vi "fyp (2) (1).vi"() -> ()   [LabVIEW 2021]
uses:
  <vilib>/userDefined/High Color/IMAQdx.ctl
  <vilib>/vision/driver/IMAQdx.llb/IMAQdx Camera Control Mode.ctl
  <vilib>/vision/driver/IMAQdx.llb/IMAQdx Acquisition Mode.ctl
  <vilib>/vision/driver/IMAQdx.llb/IMAQdx Buffer Number Mode.ctl
  <vilib>/vision/Management.llb/Cast Image 2 Method.ctl
  <vilib>/myRIO/Instrument Drivers/Onboard IO/PWM/typedefs/PWM Reference.ctl
  <vilib>/myRIO/Common/Instrument Driver Framework/Utilities/typedefs/myRIO Generic Hardware Reference.ctl
  <vilib>/myRIO/Common/Instrument Driver Framework/Utilities/typedefs/Hardware Version Enum.ctl
  <vilib>/myRIO/Common/Instrument Driver Framework/Utilities/typedefs/myRIO v1.0 Reference.ctl
  <vilib>/myRIO/Common/Instrument Driver Framework/Utilities/typedefs/Generic FPGA Reference.ctl
  <vilib>/myRIO/Common/Instrument Driver Framework/myRIO v1.0/PWM/typedefs/PWM Channels Enum.ctl
  <vilib>/myRIO/Instrument Drivers/Onboard IO/PWM/typedefs/PWM Configuration.ctl
  <vilib>/userDefined/High Color/nirio_resource_hc.ctl
  <vilib>/myRIO/Instrument Drivers/Onboard IO/DIO/typedefs/DIO Reference.ctl
  <vilib>/myRIO/Common/Instrument Driver Framework/myRIO v1.0/DIO/typedefs/DIO Channels List.ctl
  <vilib>/myRIO/Common/Instrument Driver Framework/myRIO v1.0/DIO/typedefs/DIO Channels Enum.ctl
  <vilib>/myRIO/Instrument Drivers/Onboard IO/AI/typedefs/AI Reference.ctl
  <vilib>/myRIO/Common/Instrument Driver Framework/myRIO v1.0/AI/typedefs/AI Channels List.ctl
  <vilib>/myRIO/Common/Instrument Driver Framework/myRIO v1.0/AI/typedefs/AI Channels Enum.ctl
  <vilib>/myRIO/Common/Instrument Driver Framework/Utilities/typedefs/Analog Scaling Constants List.ctl
  <vilib>/myRIO/Common/Instrument Driver Framework/Utilities/typedefs/Analog Scaling Constants.ctl
  <vilib>/myRIO/Common/Instrument Driver Framework/myRIO v1.0/DIO/vis/myRIO v1.1 Open DIO.vi
  <vilib>/myRIO/Common/Instrument Driver Framework/myRIO v1.0/PWM/vis/myRIO v1.1 Open PWM.vi
  <vilib>/myRIO/Common/Instrument Driver Framework/myRIO v1.0/AI/vis/myRIO v1.1 Open AI.vi
  <vilib>/myRIO/Common/Instrument Driver Framework/Utilities/vis/Validate Channels.vi
  <vilib>/myRIO/Common/Instrument Driver Framework/myRIO v1.0/DIO/vis/myRIO v1.0 Reserve DIO.vi
  <vilib>/myRIO/Common/Instrument Driver Framework/myRIO v1.0/PWM/vis/myRIO v1.0 Reserve PWM.vi
  <vilib>/myRIO/Instrument Drivers/Onboard IO/PWM/vis/Set Duty Cycle and Frequency.vi
  <vilib>/myRIO/Common/Instrument Driver Framework/myRIO v1.0/PWM/vis/myRIO v1.0 Close PWM.vi
  <vilib>/myRIO/Common/Instrument Driver Framework/myRIO v1.0/DIO/vis/myRIO v1.0 Close DIO.vi
  <vilib>/myRIO/Common/Instrument Driver Framework/myRIO v1.0/AI/vis/myRIO v1.0 Reserve AI.vi
  <vilib>/myRIO/Common/Instrument Driver Framework/myRIO v1.0/AI/vis/myRIO v1.0 Close AI.vi
  <vilib>/myRIO/Common/Instrument Driver Framework/myRIO v1.0/Resource Manager/vis/myRIO v1.0 Reserve Channel List.vi
  <vilib>/myRIO/Common/Instrument Driver Framework/myRIO v1.0/DIO/vis/myRIO v1.0 Build MUX Configuration DIO.vi
  <vilib>/myRIO/Common/Instrument Driver Framework/myRIO v1.0/PWM/vis/myRIO v1.0 Build MUX Configuration PWM.vi
  <vilib>/myRIO/Common/Instrument Driver Framework/myRIO v1.0/PWM/vis/myRIO v1.0 Unreserve PWM.vi
  <vilib>/myRIO/Common/Instrument Driver Framework/myRIO v1.0/DIO/vis/myRIO v1.0 Unreserve DIO.vi
  <vilib>/myRIO/Common/Instrument Driver Framework/myRIO v1.0/AI/vis/myRIO v1.0 Build MUX Configuration AI.vi
  <vilib>/myRIO/Common/Instrument Driver Framework/myRIO v1.0/AI/vis/myRIO v1.0 Unreserve AI.vi
  <vilib>/myRIO/Common/Instrument Driver Framework/myRIO v1.0/Resource Manager/vis/myRIO v1.0 Reserve Channel.vi
  <vilib>/myRIO/Common/Instrument Driver Framework/myRIO v1.0/Resource Manager/vis/myRIO v1.0 Unreserve Channel.vi
  <vilib>/myRIO/Common/Instrument Driver Framework/myRIO v1.0/Resource Manager/vis/myRIO v1.0 Create Configuration List.vi
  <vilib>/myRIO/Common/Instrument Driver Framework/myRIO v1.0/Resource Manager/vis/myRIO v1.0 Unreserve Channel List.vi
  <vilib>/myRIO/Common/Instrument Driver Framework/myRIO v1.0/Resource Manager/vis/myRIO v1.0 Build Mutex Name.vi
  <vilib>/Utility/VariantDataType/GetNumericInfo.vi
  <vilib>/Utility/error.llb/Error Cluster From Error Code.vi
  <vilib>/myRIO/Common/Instrument Driver Framework/myRIO v1.0/myRIO v1.1 Open.vi
  <vilib>/myRIO/Common/Instrument Driver Framework/myRIO v1.0/AI/vis/myRIO v1.0 Get Scaling Constants AI.vi
  <vilib>/myRIO/Common/Instrument Driver Framework/Utilities/vis/IO Manager.vi
  <vilib>/myRIO/Common/Instrument Driver Framework/Utilities/vis/Configuration Manager.vi
  <vilib>/myRIO/Common/Instrument Driver Framework/myRIO v1.0/myRIO v1.0 Close.vi
  <vilib>/myRIO/Common/Instrument Driver Framework/myRIO v1.0/Resource Manager/vis/myRIO v1.0 Configure IO.vi
  <vilib>/myRIO/Common/Instrument Driver Framework/myRIO v1.0/PWM/vis/myRIO v1.0 Write PWM.vi
  <vilib>/myRIO/Common/Instrument Driver Framework/myRIO v1.0/DIO/vis/myRIO v1.0 Read DIO.vi
  <vilib>/myRIO/Common/Instrument Driver Framework/myRIO v1.0/PWM/vis/myRIO v1.0 Shutdown PWM.vi
  <vilib>/myRIO/Common/Instrument Driver Framework/myRIO v1.0/DIO/vis/myRIO v1.0 Shutdown DIO.vi
  <vilib>/myRIO/Common/Instrument Driver Framework/myRIO v1.0/DIO/vis/myRIO v1.0 Write DIO.vi
  <vilib>/myRIO/Common/Instrument Driver Framework/myRIO v1.0/AI/vis/myRIO v1.0 Read AI.vi
  <vilib>/myRIO/Instrument Drivers/Onboard IO/AI/vis/myRIO AI Open.xnode
  <vilib>/myRIO/Instrument Drivers/Onboard IO/DIO/vis/myRIO DIO Open.xnode
  <vilib>/myRIO/Instrument Drivers/Onboard IO/PWM/vis/myRIO PWM Open.xnode
  <vilib>/vision/driver/NI_Vision_Acquisition_Software.lvlib
  <vilib>/myRIO/Instrument Drivers/Onboard IO/DIO/DIO.lvlib
  <vilib>/myRIO/Instrument Drivers/Onboard IO/AI/AI.lvlib
  <vilib>/myRIO/Instrument Drivers/Onboard IO/PWM/PWM.lvlib
  <vilib>/vision/NI_Vision_Development_Module.lvlib
panel:
  out "error out 2":errorcluster
  in  "LED0":bool
  out "Image 2":T1(plugin-control)
  in  "Session In 2":T2
  out "Colour Match Score 2":i32[](array[numeric])
  out "Is Colour from Sample Detected 2":bool
  out "Number of Circles Returned 2":i32
  out "Boolean 4":bool
  in  "error in (no error)":errorcluster
  out "Boolean 2":bool
  in  "error in (no error) 3":errorcluster
  in  "error in (no error) 2":errorcluster
  out "error out":errorcluster
  out "Darkness level":dbl(slide) scale=0.0..1.0
  out "Numeric":dbl format="%.2f"
  out "Image":T1(plugin-control)
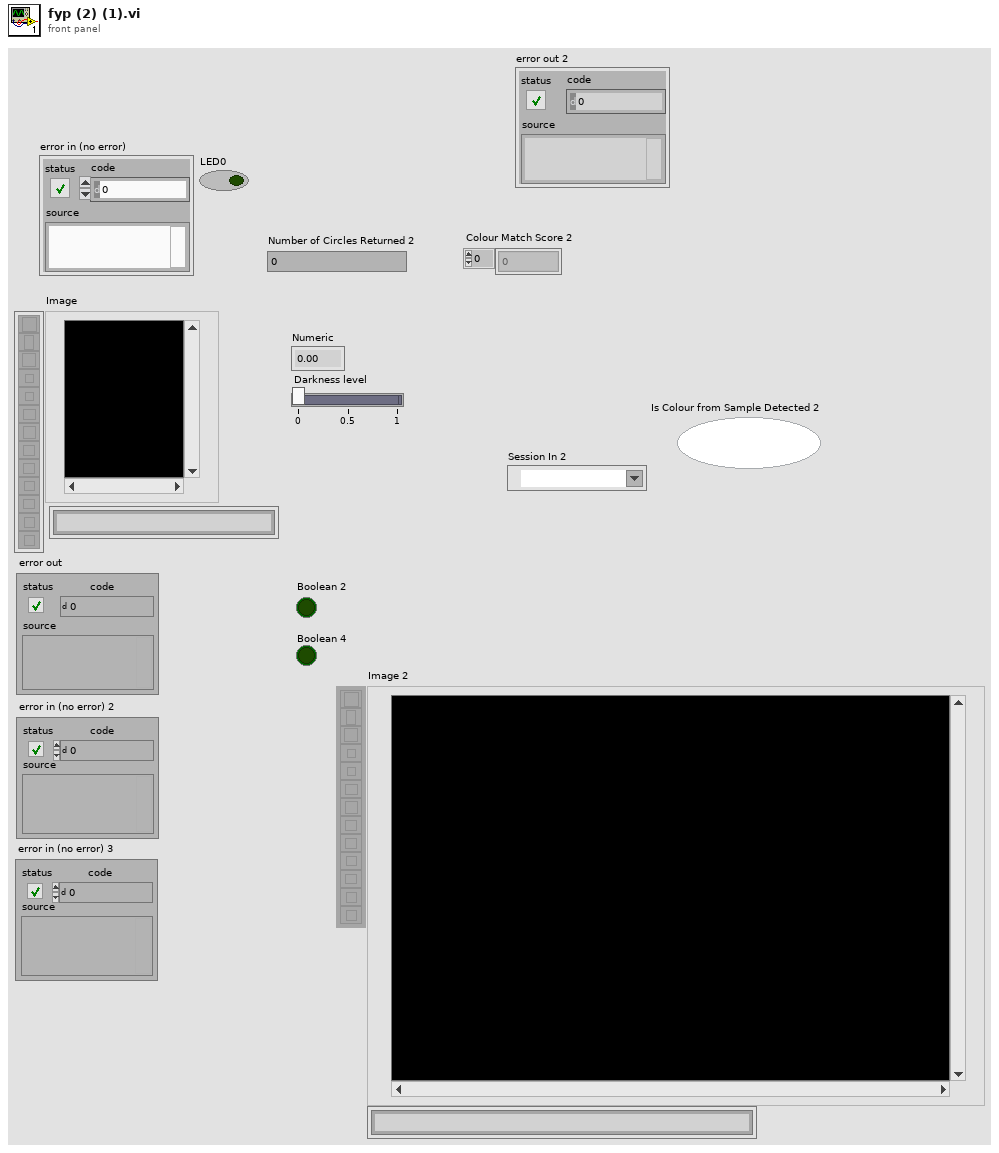
[diagram p1: front panel]
types:
  T1 = typedef "IMAQ Image.ctl" = refnum<image>
  T2 = typedef "IMAQdx.ctl" = refnum<k21>
  T3 = typedef "Cast Image 2 Method.ctl" = u32
  T4 = typedef "Image Type" = u32
  T5 = typedef "IMAQ Rectangle" = cluster{"Left":i32, "Top":i32, "Right":i32, "Bottom":i32, "Rotation":dbl}
  T6 = typedef "NI_Vision_Acquisition_Software.lvlib/IMAQdx Buffer Number Mode.ctl" = enum32{"Next", "Last", "Buffer Number", "Every", "Last New"}
  T7 = typedef "NI_Vision_Acquisition_Software.lvlib/IMAQdx Acquisition Mode.ctl" = enum32{"One Shot", "Continuous"}
  T8 = typedef "NI_Vision_Acquisition_Software.lvlib/IMAQdx Camera Control Mode.ctl" = enum32{"Controller", "Listener"}
  T9 = typedef "DIO.lvlib/DIO Reference.ctl" = cluster{"myRIO Reference":T10, "DIO Channels List":T14}
  T10 = typedef "myRIO Generic Hardware Reference.ctl" = cluster{"myRIO Model":T11, "myRIO Hardware Reference":T12}
  T11 = typedef "Hardware Version Enum.ctl" = enum16{"Unknown", "myRIO-1900", "myRIO-1950", "roboRIO", "NI ELVIS RIO CM", "ELVIS III"}
  T12 = typedef "myRIO v1.0 Reference.ctl" = cluster{"Generic FPGA Reference":T13, "Allow multiple opens":bool}
  T13 = typedef "Generic FPGA Reference.ctl" = refnum<k20>
  T14 = typedef "DIO Channels List.ctl" = T15[]
  T15 = typedef "DIO Channels Enum.ctl" = enum16{"Not Connected", "C/DIO0", "C/DIO1", "C/DIO2", "C/DIO3", "C/DIO4", "C/DIO5", "C/DIO6", "C/DIO7", "A/DIO0", "A/DIO1", "A/DIO2", "A/DIO3", "A/DIO4", "A/DIO5", "A/DIO6", "A/DIO7", "A/DIO8", "A/DIO9", "A/DIO10", "A/DIO11", "A/DIO12", "A/DIO13", "A/DIO14", "A/DIO15", "A/DIO16", "A/DIO17", "A/DIO18", "A/DIO19", "B/DIO0", "B/DIO1", "B/DIO2", "B/DIO3", "B/DIO4", "B/DIO5", "B/DIO6", "B/DIO7", "B/DIO8", "B/DIO9", "B/DIO10", "B/DIO11", "B/DIO12", "B/DIO13", "B/DIO14", "B/DIO15", "B/DIO16", "B/DIO17", "B/DIO18", "B/DIO19", "LED0", "LED1", "LED2", "LED3", "Button0", "DIO/DIO0", "DIO/DIO1", "DIO/DIO2", "DIO/DIO3", "DIO/DIO4", "DIO/DIO5", "DIO/DIO6", "DIO/DIO7", "DIO/DIO8", "DIO/DIO9", "SPI/CS0", "SPI/CS1", "SPI/CS2", "SPI/CS3", "LED RADIO (Green)", "LED RADIO (Red)", "LED COMM (Green)", "LED COMM (Red)", "LED MODE (Green)", "LED MODE (Red)"}
  T16 = typedef "PWM.lvlib/PWM Reference.ctl" = cluster{"myRIO Reference":T10, "PWM Channels Enum":T17, "PWM Configuration":T18}
  T17 = typedef "PWM Channels Enum.ctl" = enum16{"Not Connected", "C/PWM0", "C/PWM1", "A/PWM0", "A/PWM1", "A/PWM2", "A/PWM3", "A/PWM4", "A/PWM5", "A/PWM6", "A/PWM7", "A/PWM8", "A/PWM9", "A/PWM10", "A/PWM11", "A/PWM12", "A/PWM13", "A/PWM14", "A/PWM15", "A/PWM16", "A/PWM17", "A/PWM18", "A/PWM19", "B/PWM0", "B/PWM1", "B/PWM2", "B/PWM3", "B/PWM4", "B/PWM5", "B/PWM6", "B/PWM7", "B/PWM8", "B/PWM9", "B/PWM10", "B/PWM11", "B/PWM12", "B/PWM13", "B/PWM14", "B/PWM15", "B/PWM16", "B/PWM17", "B/PWM18", "B/PWM19", "PWM/PWM0", "PWM/PWM1", "PWM/PWM2", "PWM/PWM3", "PWM/PWM4", "PWM/PWM5", "PWM/PWM6", "PWM/PWM7", "PWM/PWM8", "PWM/PWM9"}
  T18 = typedef "PWM.lvlib/PWM Configuration.ctl" = cluster{"Frequency":dbl, "Duty Cycle":dbl}
  T19 = typedef "AI.lvlib/AI Reference.ctl" = cluster{"myRIO Reference":T10, "AI Channels List":T20, "AI Scaling Constants List":T22}
  T20 = typedef "AI Channels List.ctl" = T21[]
  T21 = typedef "AI Channels Enum.ctl" = enum16{"Not Connected", "AudioIn/Left", "AudioIn/Right", "C/AI0", "C/AI1", "A/AI0", "A/AI1", "A/AI2", "A/AI3", "A/AI4", "A/AI5", "A/AI6", "A/AI7", "B/AI0", "B/AI1", "B/AI2", "B/AI3", "B/AI4", "B/AI5", "B/AI6", "B/AI7", "AI/AI0", "AI/AI1", "AI/AI2", "AI/AI3", "A/AI0 (DIFF)", "A/AI1 (DIFF)", "A/AI2 (DIFF)", "A/AI3 (DIFF)", "B/AI0 (DIFF)", "B/AI1 (DIFF)", "B/AI2 (DIFF)", "B/AI3 (DIFF)"}
  T22 = typedef "Analog Scaling Constants List.ctl" = T23[]
  T23 = typedef "Analog Scaling Constants.ctl" = cluster{"LSB Weight (Volts)":dbl, "Offset (Volts)":dbl, "Signed?":bool}
  T24 = typedef "ROI Descriptor" = cluster{"Global Rectangle":i32[], "Contours":cluster{"ID":enum32{"External", "Internal"}, "Type":u32, "Coordinates":i32[]}[]}
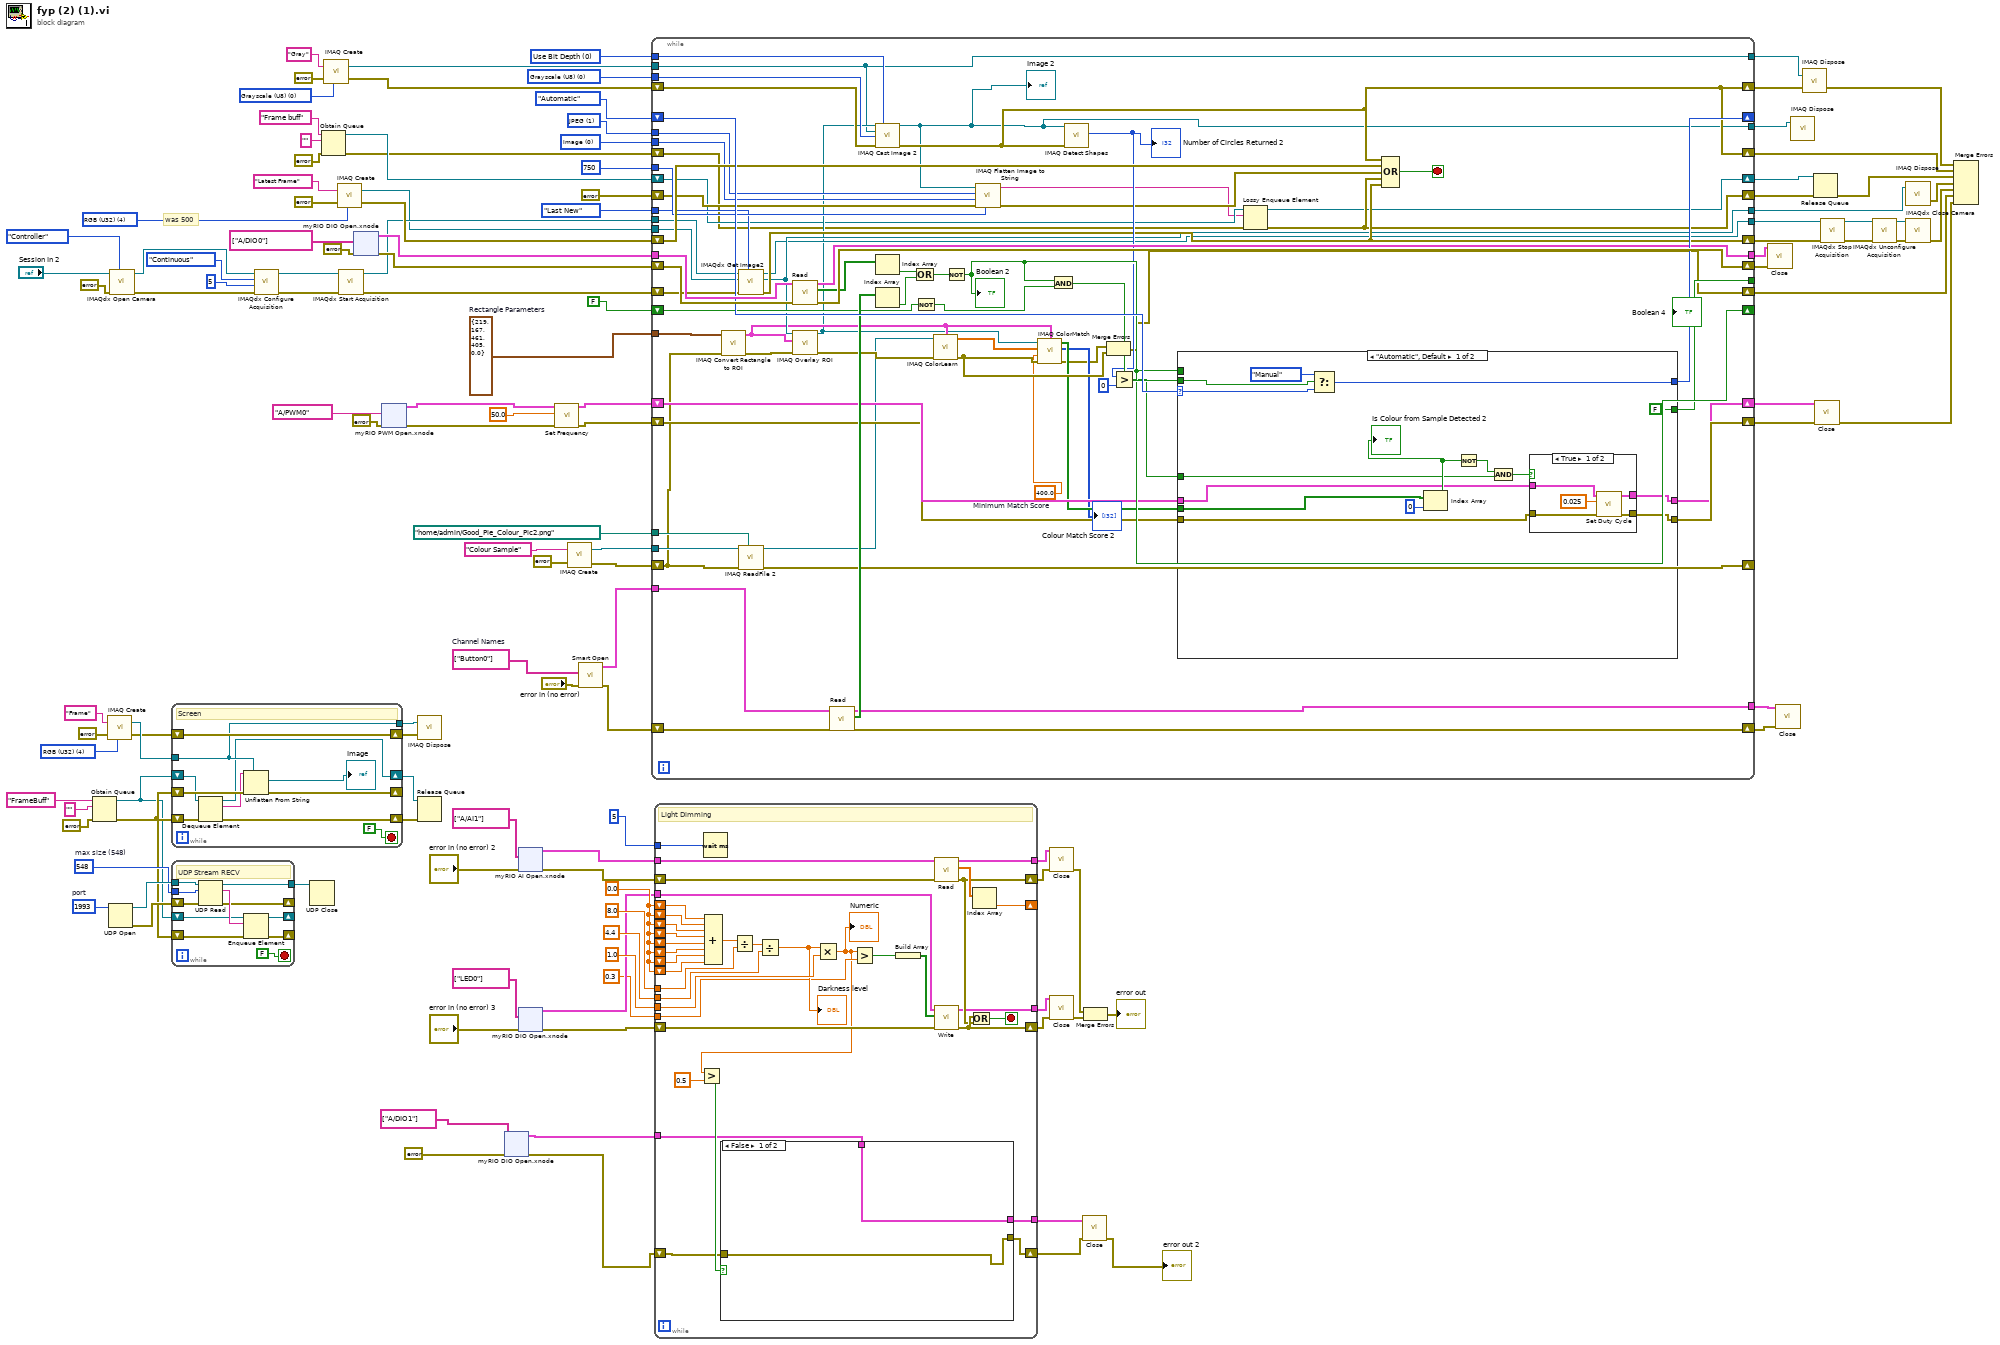
[diagram p0: block diagram]
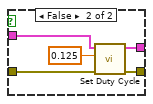
[diagram p2: hidden frame]
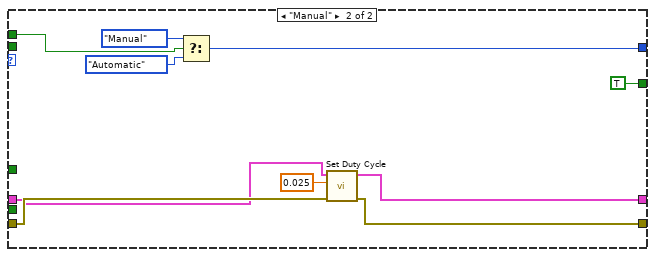
[diagram p3: hidden frame]
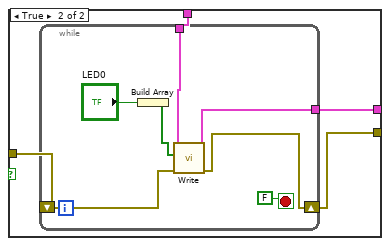
[diagram p4: hidden frame]
diagram:
  w51 = T3 0 items=["Use Bit Depth", "Shift", "Use Lookup Table"] ("Method")
  w50 = T4 0 items=["Grayscale (U8)", "Grayscale (I16)", "Grayscale (SGL)", "Complex (CSG)", "RGB (U32)", "HSL (U32)", "RGB (U64)", "Grayscale (U16)"] ("Image Type")
  w39 = T5 {"Left"=219, "Top"=167, "Right"=461, "Bottom"=405, "Rotation"=0.0}  # Rectangle Parameters
  w47 = 0 items=["Image", "Image and Vision Info", "Reference to Image"] ("Type of Flatten (Image and Vision Info)")
  w48 = 1 items=["None", "JPEG", "PACKED BINARY"] ("Compression (None)")
  w74 = T4 4 items=["Grayscale (U8)", "Grayscale (I16)", "Grayscale (SGL)", "Complex (CSG)", "RGB (U32)", "HSL (U32)", "RGB (U64)", "Grayscale (U16)"] ("Image Type")
  w75 = T4 0 items=["Grayscale (U8)", "Grayscale (I16)", "Grayscale (SGL)", "Complex (CSG)", "RGB (U32)", "HSL (U32)", "RGB (U64)", "Grayscale (U16)"] ("Image Type")
  w85 = tag[] ["Button0"]  # Channel Names
  w105 = 0.0
  w114 = 548  # max size (548)
  w117 = u16 1993  # port
  w126 = T4 4 items=["Grayscale (U8)", "Grayscale (I16)", "Grayscale (SGL)", "Complex (CSG)", "RGB (U32)", "HSL (U32)", "RGB (U64)", "Grayscale (U16)"] ("Image Type")
  # "was 500"
  n1 = Obtain Queue(name (unnamed)="FrameBuff", element data type="", error in (no error)=errorcluster {"status"=FALSE, "code"=0, "source"=""}) -> (queue out=w111:refnum<queue>, error out=w113:errorcluster)  [unwired: 2 in, 1 out]
  n2 = call "IMAQ Create"("Image Name"="Frame", "Image Type"=w126, "error in (no error)"=errorcluster {"status"=FALSE, "code"=0, "source"=""}) -> ("New Image"=w123:T1, "error out"=w112:errorcluster)  [unwired: 2 in]
  n3 = UDP Open(11:w117) -> (port=w115:refnum<k16>, 0:w116:errorcluster)  [unwired: 4 in, 1 out]
  n4 = call <vilib>:"IMAQdx Open Camera.vi"("Camera Control Mode"=IMAQdx_Camera_Control_Mode."Controller", "error in"=errorcluster {"status"=FALSE, "code"=0, "source"=""}, "Session In"="Session In 2") -> ("error out"=w73:errorcluster, "Session Out"=w70:T2)  [unwired: 7 in]
  n5 = while {
    shift-right: [w136] -> w122
    shift-left: w112 -> [w136]
    shift-right: [w134] -> w120
    shift-left: w113 -> [w138]
    shift-right: [w133] -> w119
    shift-left: w111 -> [w137]
    shift-right: [w130] -> _
    shift-left: w113 -> [w139]
    tunnel: w123 -> [w135]
    tunnel: [w135] -> w121
    stop <- FALSE stop-if-true
    # "Screen"
    n6 = Dequeue Element(queue=w137, error in (no error)=w138) -> (queue out=w133:refnum<queue>, element=w132:string, error out=w134:errorcluster)  [unwired: 1 in, 1 out]
    n7 = Unflatten From String(type=w135, binary string=w132, error in (no error)=w139) -> (value=→"Image":T1, error out=w130:errorcluster)  [unwired: 2 in, 1 out]
  }
  n8 = while {
    shift-right: [w140] -> _
    shift-left: w116 -> [w150]
    tunnel: w115 -> [w149]
    tunnel: w114 -> [w148]
    shift-right: [w146] -> _
    shift-left: w113 -> [w143]
    shift-right: [w147] -> _
    shift-left: w111 -> [w144]
    tunnel: [w142] -> w110
    stop <- FALSE stop-if-true
    # "UDP Stream RECV"
    n9 = UDP Read(connection ID=w149, max size (548)=w148, 8:w150) -> (data out=w145:string, error out=w140:errorcluster, 3:w142:refnum<k16>)  [unwired: 1 in, 2 out]
    n10 = Enqueue Element(queue=w144, element=w145, error in (no error)=w143) -> (queue out=w147:refnum<queue>, error out=w146:errorcluster)  [unwired: 1 in, 1 out]
  }
  n11 = call <vilib>:"IMAQdx Configure Acquisition.vi"("error in"=w73, "Number of Buffers"=u32 5, "Continuous?"=IMAQdx_Acquisition_Mode."Continuous", "Session In"=w70) -> ("error out"=w72:errorcluster, "Session Out"=w69:T2)  [unwired: 6 in]
  n12 = UDP Close(connection ID=w110) -> ()  [unwired: 1 in, 2 out]
  n13 = Obtain Queue(name (unnamed)="Frame buff", element data type="", error in (no error)=errorcluster {"status"=FALSE, "code"=0, "source"=""} ("error in")) -> (queue out=w45:refnum<queue>, error out=w44:errorcluster)  [unwired: 2 in, 1 out]
  n14 = call "IMAQ Create"("Image Name"="Gray", "Image Type"=w75, "error in (no error)"=errorcluster {"status"=FALSE, "code"=0, "source"=""}) -> ("New Image"=w49:T1, "error out"=w14:errorcluster)  [unwired: 2 in]
  n15 = call "IMAQ Create"("Image Name"="Latest Frame", "Image Type"=w74, "error in (no error)"=errorcluster {"status"=FALSE, "code"=0, "source"=""} ("error in")) -> ("New Image"=w40:T1, "error out"=w43:errorcluster)  [unwired: 2 in]
  n16 = call <vilib>:"IMAQdx Start Acquisition.vi"("error in"=w72, "Session In"=w69) -> ("error out"=w42:errorcluster, "Session Out"=w41:T2)  [unwired: 8 in]
  n17 = xnode ("myRIO DIO Open.xnode")("error in (no error)"=errorcluster {"status"=FALSE, "code"=0, "source"=""}, "Channel Names"=tag[] ["A/DIO0"]) -> ("error out"=w86:errorcluster, "DIO Ref Out"=w78:T9)  [unwired: 1 in]
  n18 = xnode "myRIO PWM Open.xnode"("error in (no error)"=errorcluster {"status"=FALSE, "code"=0, "source"=""}, "Channel Name"=tag "A/PWM0") -> ("error out"=w53:errorcluster, "PWM Ref Out"=w54:T16)  [unwired: 1 in]
  n19 = call "IMAQ Dispose"("Image"=w121, "error in (no error)"=w122) -> ()  [unwired: 4 in, 1 out]
  n20 = Release Queue(queue=w119, error in (no error)=w120) -> ()  [unwired: 1 in, 3 out]
  n21 = xnode "myRIO DIO Open.xnode"("error in (no error)"=errorcluster {"status"=FALSE, "code"=0, "source"=""}, "Channel Names"=tag[] ["A/DIO1"]) -> ("error out"=w5:errorcluster, "DIO Ref Out"=w7:T9)  [unwired: 1 in]
  n22 = xnode "myRIO AI Open.xnode"("error in (no error)"="error in (no error) 2", "Channel Names"=tag[] ["A/AI1"]) -> ("error out"=w108:errorcluster, "AI Ref Out"=w109:T19)  [unwired: 1 in]
  n23 = xnode "myRIO DIO Open.xnode"("error in (no error)"="error in (no error) 3", "Channel Names"=tag[] ["LED0"]) -> ("error out"=w99:errorcluster, "DIO Ref Out"=w100:T9)  [unwired: 1 in]
  n24 = call <vilib>:"Set Frequency.vi"("error in (no error)"=w53, "Frequency [Hz]"=50.0, "PWM Ref In"=w54) -> ("error out"=w36:errorcluster, "PWM Ref Out"=w37:T16)  [unwired: 6 in]
  n25 = call "IMAQ Create"("Image Name"="Colour Sample", "error in (no error)"=errorcluster {"status"=FALSE, "code"=0, "source"=""}) -> ("New Image"=w38:T1, "error out"=w9:errorcluster)  [unwired: 3 in]
  n26 = call <vilib>:"Smart Open.vi"("error in (no error)"="error in (no error)", "Channel Names"=w85) -> ("error out"=w88:errorcluster, "DIO Ref Out"=w20:T9)  [unwired: 8 in]
  n27 = while {
    shift-right: [w216] -> w81
    shift-left: w88 -> [w217]
    shift-right: [w215] -> w80
    shift-left: w86 -> [w219]
    tunnel: w78 -> [w218]
    shift-right: [w212] -> _
    shift-left: enum16{"Automatic", "Manual"}."Automatic" -> [w214]
    tunnel: [w211] -> w82
    shift-right: [w203] -> _
    shift-left: FALSE -> [w208]
    tunnel: [w202] -> _
    tunnel: w51 -> [w193]
    tunnel: w50 -> [w192]
    tunnel: w49 -> [w164]
    tunnel: w48 -> [w186]
    tunnel: w47 -> [w187]
    tunnel: 750 ("Quality (750)") -> [w189]
    tunnel: w41 -> [w181]
    tunnel: w40 -> [w182]
    tunnel: w39 -> [w174]
    tunnel: w38 -> [w176]
    tunnel: path "/home/admin/Good_Pie_Colour_Pic2.png" ("File Path") -> [w177]
    tunnel: [w179] -> w25
    tunnel: [w178] -> w24
    tunnel: IMAQdx_Buffer_Number_Mode."Last New" ("Buffer Number Mode (Next)") -> [w184]
    tunnel: [w164] -> w22
    shift-right: [w197] -> w21
    shift-left: w36 -> [w200]
    tunnel: [w196] -> w18
    tunnel: w20 -> [w195]
    shift-right: [w194] -> w19
    shift-left: w37 -> [w201]
    shift-right: [w165] -> w10
    shift-left: w45 -> [w169]
    shift-right: [w180] -> w16
    shift-left: w43 -> [w199]
    shift-right: [w153] -> w17
    shift-left: w42 -> [w183]
    shift-right: [w175] -> _
    shift-left: w9 -> [w162]
    shift-right: [w161] -> w15
    shift-left: w14 -> [w191]
    shift-right: [w161] -> w13
    shift-left: w44 -> [w167]
    shift-right: [w166] -> w12
    shift-left: errorcluster {"status"=FALSE, "code"=0, "source"=""} ("error in") -> [w188]
    tunnel: [w151] -> w8
    stop <- w198 stop-if-true
    w157 = 400.0  # Minimum Match Score
    n28 = call "IMAQ Convert Rectangle to ROI"("error in (no error)"=w162, "Rectangle"=w174) -> ("error out"=w172:errorcluster, "ROI Descriptor"=w173:T24)  [unwired: 7 in]
    n29 = call <vilib>:"IMAQdx Get Image2.vi"("Buffer Number Mode (Next)"=w184, "error in"=w183, "Image In"=w182, "Session In"=w181) -> ("error out"=w180:errorcluster, "Image Out"=w179:T1, "Session Out"=w178:T2)  [unwired: 4 in, 1 out]
    n30 = call "IMAQ ReadFile 2"("File Path"=w177, "error in (no error)"=w162, "Image"=w176) -> ("error out"=w175:errorcluster, "Image Out"=w160:T1)  [unwired: 4 in, 3 out]
    n31 = call <vilib>:"Read.vi"("error in (no error)"=w219, "DIO Ref In"=w218) -> ("error out"=w215:errorcluster, "Values"=w206:bool[], "DIO Ref Out"=w211:T9)  [unwired: 7 in]
    n32 = call "IMAQ Overlay ROI"("error in (no error)"=w172, "ROI Descriptor"=w173, "Image"=w179) -> ("error out"=w171:errorcluster, "Image Out"=w170:T1)  [unwired: 7 in]
    n33 = call <vilib>:"Read.vi"("error in (no error)"=w217, "DIO Ref In"=w195) -> ("error out"=w216:errorcluster, "Values"=w213:bool[], "DIO Ref Out"=w196:T9)  [unwired: 7 in]
    n34 = call "IMAQ Cast Image 2"("Image Src"=w170, "Method"=w193, "Image Dst"=w164, "Image Type"=w192, "error in (no error)"=w191) -> ("Image Dst Out"=w151:T1, "error out"=w161:errorcluster)  [unwired: 9 in]
    "Image 2" <- w151
    n35 = Index Array(array=w206) -> (element=w209:bool)  [unwired: 1 in]
    n36 = Index Array(array=w213) -> (element=w210:bool)  [unwired: 1 in]
    n37 = Or(x=w209, y=w210) -> (x .or. y?=w205:bool)
    n38 = Not(x=w208) -> (.not. x?=w207:bool)
    n39 = call "IMAQ ColorLearn"("ROI Descriptor"=w173, "Image"=w160, "error in (no error)"=w171) -> ("Color Spectrum"=w158:dbl[], "error out"=w159:errorcluster)  [unwired: 5 in]
    n40 = Not(x=w205) -> (.not. x?=w203:bool)
    "Boolean 2" <- w203
    n41 = call "IMAQ Flatten Image to String"("Quality (750)"=w189, "error in (no error)"=w188, "Type of Flatten (Image and Vision Info)"=w187, "Compression (None)"=w186, "Image"=w151) -> ("error out"=w185:errorcluster, "Data String"=w168:string)  [unwired: 5 in]
    n42 = call "IMAQ ColorMatch"("ROI Descriptor"=w173, "Image"=w170, "Color Spectrum"=w158, "Minimum Match Score"=w157, "error in (no error)"=w159) -> ("Match Flag"=w156:bool[], "Match Score"=→"Colour Match Score 2":i32[], "error out"=w154:errorcluster)  [unwired: 2 in]
    n43 = And(x=w203, y=w207) -> (x .and. y?=w204:bool)
    n44 = call-poly "IMAQ Detect Shapes"("error in (no error)"=w161, "Image"=w151) -> ("Number of Matches Returned"=w190:i32)  [unwired: 7 in, 2 out]
    "Number of Circles Returned 2" <- w190
    n45 = Merge Errors(w154, w159) -> (w153:errorcluster)
    n46 = Greater?(x=w190, y=0) -> (0:w152:bool)
    n47 = case shown="\"Automatic\", Default" w214 {
      selector: w214 -> [w232 _]
      tunnel: [w233 w250] -> w212
      tunnel: w204 -> [w231 _]
      tunnel: [FALSE TRUE] -> w202
      tunnel: w203 -> [_ w251]
      tunnel: w201 -> [w226 w247]
      tunnel: w200 -> [w225 w248]
      tunnel: [w224 w245] -> w194
      tunnel: [w223 w246] -> w197
      tunnel: w152 -> [w221 _]
      tunnel: w156 -> [w220 _]
      frame "Automatic", Default {
        n48 = Select(t=enum16{"Automatic", "Manual"}."Manual", s=w231, f=w232) -> (s? t:f=w233:enum16{"Automatic", "Manual"})
        n49 = Index Array(array=w220, index=0) -> (element=w227:bool)
        "Is Colour from Sample Detected 2" <- w227
        n50 = Not(x=w227) -> (.not. x?=w228:bool)
        n51 = And(x=w228, y=w221) -> (x .and. y?=w222:bool)
        n52 = case shown="True" w222 {
          tunnel: w225 -> [w238 w242]
          tunnel: [w237 w241] -> w223
          tunnel: w226 -> [w239 w244]
          tunnel: [w236 w240] -> w224
          frame True {
            n53 = call <vilib>:"Set Duty Cycle.vi"("error in (no error)"=w238, "Duty Cycle"=0.025, "PWM Ref In"=w239) -> ("error out"=w237:errorcluster, "PWM Ref Out"=w236:T16)  [unwired: 6 in]
          }
          frame False {
            n54 = call <vilib>:"Set Duty Cycle.vi"("error in (no error)"=w242, "Duty Cycle"=0.125, "PWM Ref In"=w244) -> ("error out"=w241:errorcluster, "PWM Ref Out"=w240:T16)  [unwired: 6 in]
          }
        }
      }
      frame "Manual" {
        n55 = Select(t=enum16{"Automatic", "Manual"}."Manual", s=w251, f=enum16{"Automatic", "Manual"}."Automatic") -> (s? t:f=w250:enum16{"Automatic", "Manual"})
        n56 = call <vilib>:"Set Duty Cycle.vi"("error in (no error)"=w248, "Duty Cycle"=0.025, "PWM Ref In"=w247) -> ("error out"=w246:errorcluster, "PWM Ref Out"=w245:T16)  [unwired: 6 in]
      }
    }
    "Boolean 4" <- w202
    n57 = Lossy Enqueue Element(queue=w169, element=w168, error in (no error)=w167) -> (queue out=w165:refnum<queue>, error out=w166:errorcluster)  [unwired: 2 out]
    n58 = Compound Arithmetic op=OR(w161, w199, w185, w166, w180) -> (w198:bool)
  }
  n59 = while {
    tunnel: w109 -> [w290]
    shift-right: [w267] -> w107
    shift-left: w108 -> [w289]
    tunnel: [w288] -> w106
    shift-right: [w278] -> _
    shift-left: w105 -> [w280]
    shift-left: w105 -> [w281]
    shift-left: w105 -> [w282]
    shift-left: w105 -> [w283]
    shift-left: w105 -> [w284]
    shift-left: w105 -> [w285]
    shift-left: w105 -> [w286]
    shift-left: w105 -> [w287]
    tunnel: 8.0 -> [w277]
    tunnel: u32 5 ("millisecond timer value") -> [w275]
    tunnel: 4.4 -> [w274]
    tunnel: 1.0 -> [w272]
    tunnel: w100 -> [w270]
    shift-right: [w268] -> w98
    shift-left: w99 -> [w269]
    tunnel: [w266] -> w97
    tunnel: 0.3 ("y") -> [w264]
    tunnel: w7 -> [w258]
    shift-right: [w255] -> w2
    shift-left: w5 -> [w257]
    tunnel: [w256] -> w3
    stop <- w265 stop-if-true
    # "Light Dimming"
    n60 = Wait (ms)(milliseconds to wait=w275) -> ()  [unwired: 1 out]
    n61 = Compound Arithmetic op=ADD(w280, w281, w282, w283, w284, w285, w286, w287) -> (w276:dbl)
    n62 = Divide(x=w276, y=w277) -> (x/y=w273:dbl)
    n63 = Divide(x=w273, y=w274) -> (x/y=w271:dbl)
    "Darkness level" <- w271
    n64 = Multiply(x=w271, y=w272) -> (x*y=w261:dbl)
    "Numeric" <- w261
    n65 = Greater?(x=w261, y=0.5) -> (0:w259:bool)
    n66 = case shown="False" w259 {
      tunnel: w257 -> [w292 w296]
      tunnel: w258 -> [w291 w295]
      tunnel: [w292 w294] -> w255
      tunnel: [w291 w293] -> w256
      frame False {
      }
      frame True {
        n67 = while {
          tunnel: w295 -> [w300]
          shift-right: [w298] -> w294
          shift-left: w296 -> [w301]
          tunnel: [w299] -> w293
          stop <- FALSE stop-if-true
          n68 = Build Array("LED0") -> (w302:bool[])
          n69 = call <vilib>:"Write.vi"("error in (no error)"=w301, "Values"=w302, "DIO Ref In"=w300) -> ("error out"=w298:errorcluster, "DIO Ref Out"=w299:T9)  [unwired: 6 in]
        }
      }
    }
    n70 = Greater?(x=w261, y=w264) -> (0:w263:bool)
    n71 = Build Array(w263) -> (w262:bool[])
    n72 = call <vilib>:"Read.vi"("error in (no error)"=w289, "AI Ref In"=w290) -> ("error out"=w267:errorcluster, "Values"=w279:dbl[], "AI Ref Out"=w288:T19)  [unwired: 7 in]
    n73 = call <vilib>:"Write.vi"("error in (no error)"=w269, "Values"=w262, "DIO Ref In"=w270) -> ("error out"=w268:errorcluster, "DIO Ref Out"=w266:T9)  [unwired: 6 in]
    n74 = Or(x=w268, y=w267) -> (x .or. y?=w265:bool)
    n75 = Index Array(array=w279) -> (element=w278:dbl)  [unwired: 1 in]
  }
  n76 = call <vilib>:"Close.vi"("error in (no error)"=w107, "AI Ref In"=w106) -> ("error out"=w95:errorcluster)  [unwired: 9 in]
  n77 = call <vilib>:"Close.vi"("error in (no error)"=w98, "DIO Ref In"=w97) -> ("error out"=w94:errorcluster)  [unwired: 9 in]
  n78 = call <vilib>:"Close.vi"("error in (no error)"=w2, "DIO Ref In"=w3) -> ("error out"=→"error out 2":errorcluster)  [unwired: 9 in]
  n79 = Merge Errors(w95, w94) -> (→"error out":errorcluster)
  n80 = call <vilib>:"Close.vi"("error in (no error)"=w80, "DIO Ref In"=w82) -> ()  [unwired: 9 in, 1 out]
  n81 = call <vilib>:"Close.vi"("error in (no error)"=w81, "DIO Ref In"=w18) -> ()  [unwired: 9 in, 1 out]
  n82 = call "IMAQ Dispose"("Image"=w8) -> ()  [unwired: 5 in, 1 out]
  n83 = call "IMAQ Dispose"("Image"=w22, "error in (no error)"=w15) -> ("error out"=w26:errorcluster)  [unwired: 4 in]
  n84 = Release Queue(queue=w10, error in (no error)=w12) -> (error out=w28:errorcluster)  [unwired: 1 in, 2 out]
  n85 = call <vilib>:"Close.vi"("error in (no error)"=w21, "PWM Ref In"=w19) -> ("error out"=w27:errorcluster)  [unwired: 9 in]
  n86 = call <vilib>:"IMAQdx Stop Acquisition.vi"("error in"=w16, "Session In"=w24) -> ("error out"=w32:errorcluster, "Session Out"=w31:T2)  [unwired: 8 in]
  n87 = call <vilib>:"IMAQdx Unconfigure Acquisition.vi"("error in"=w32, "Session In"=w31) -> ("error out"=w34:errorcluster, "Session Out"=w33:T2)  [unwired: 8 in]
  n88 = call "IMAQ Dispose"("Image"=w25) -> ("error out"=w29:errorcluster)  [unwired: 5 in]
  n89 = call <vilib>:"IMAQdx Close Camera.vi"("error in"=w34, "Session In"=w33) -> ("error out"=w30:errorcluster)  [unwired: 9 in]
  n90 = Merge Errors(w26, w13, w28, w29, w30, w17, w27) -> ()  [unwired: 1 out]
